vi "PID Movement final version.vi"(2 "error in (no error)":errorcluster, 3 "Yaw":dbl, 4 "Speed":dbl, 5 "Direction":T1) -> (0 "error out":errorcluster, 1 "Speed & distance":T2)   [LabVIEW 2018]
uses:
  PID Movement final version Type Def.ctl
  <vilib>/Studica/Studica Toolkit/Background/Mxp Selection.ctl
  <vilib>/addons/control/pid/pid.llb/PID (DBL).vi
  <vilib>/addons/control/pid/NI_PID_pid.lvlib
panel:
  out "Vx":dbl
  out "M2":dbl
  out "M1":dbl
  out "M0":dbl
  out "S2":dbl
  out "S1":dbl
  out "S0":dbl
  out "M2 Distance":dbl
  out "M1 Distance":dbl
  out "M0 Distance":dbl
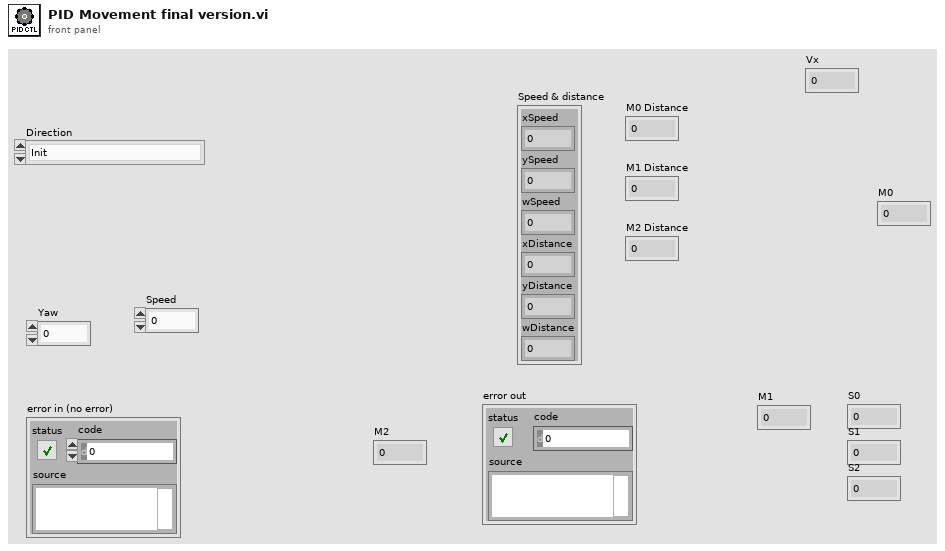
[diagram p1: front panel]
types:
  T1 = typedef "PID Movement final version Type Def.ctl" = enum16{"Init", "Front Back", "Left Right", "Rotate", "Latch", "Stop"}
  T2 = cluster{"xSpeed":dbl, "ySpeed":dbl, "wSpeed":dbl, "xDistance":dbl, "yDistance":dbl, "wDistance":dbl}
  T3 = cluster{"proportional gain (Kc)":dbl, "integral time (Ti, min)":dbl, "derivative time (Td, min)":dbl}
  T4 = typedef "Mxp Selection.ctl" = enum16{"MXP A", "MXP B"}
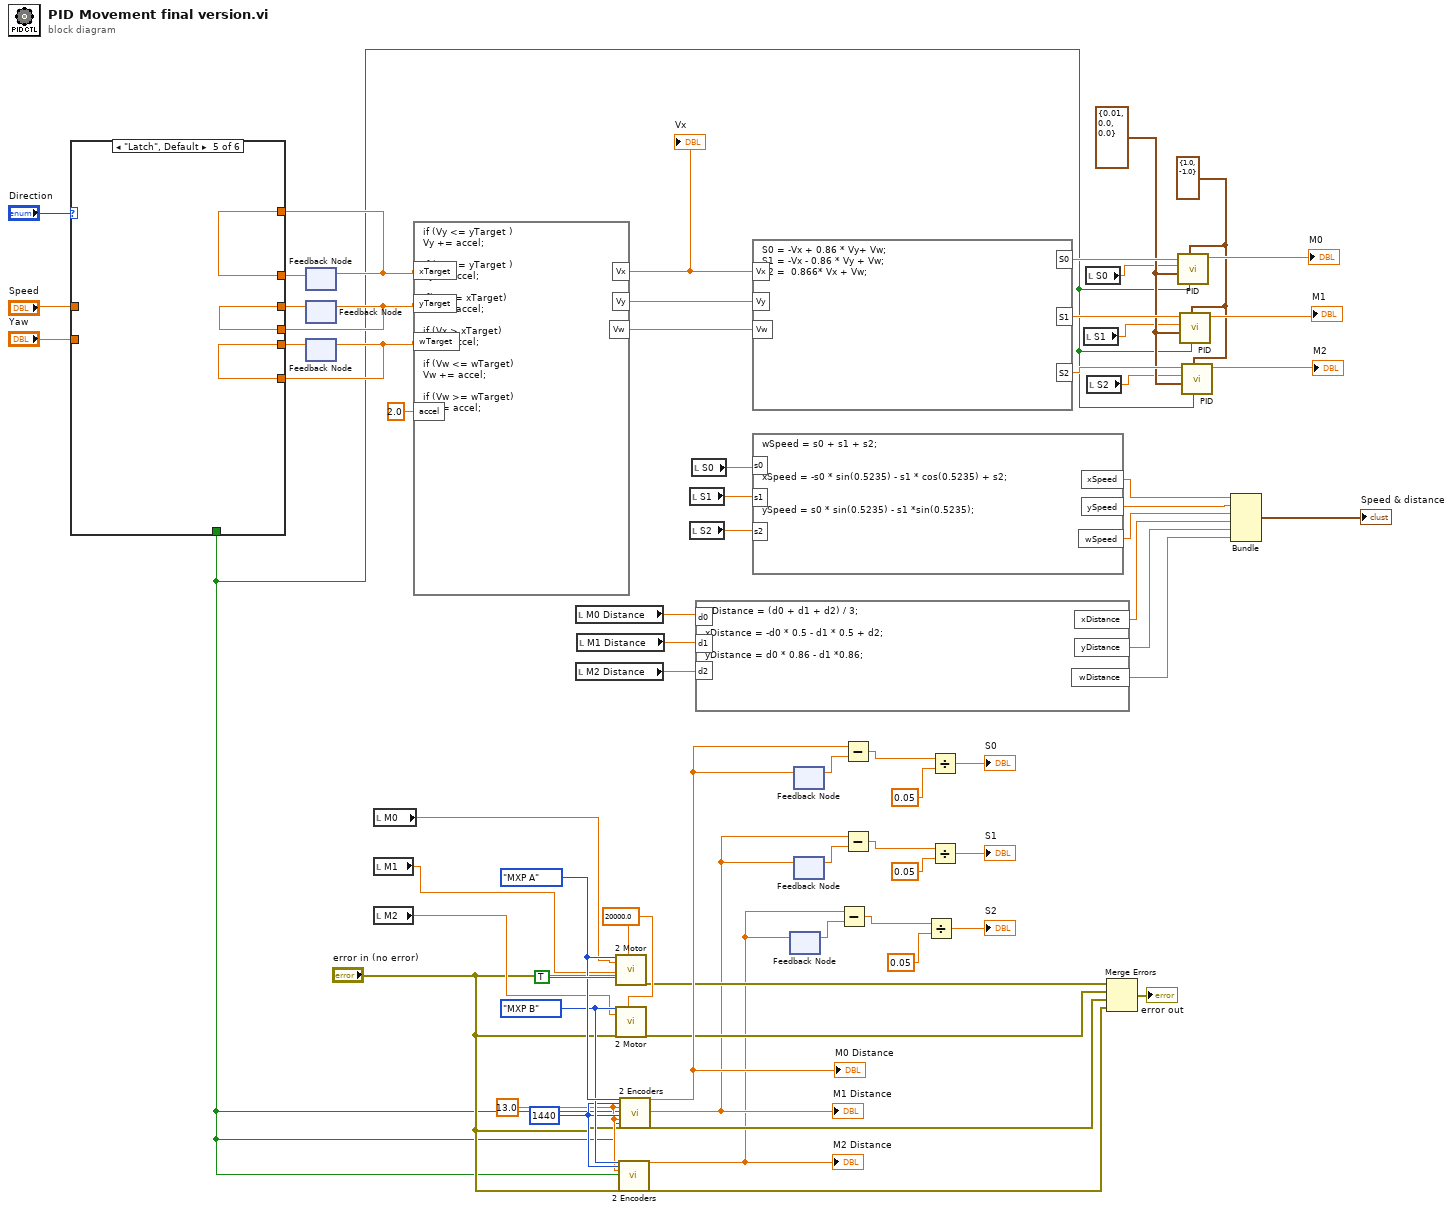
[diagram p0: block diagram]
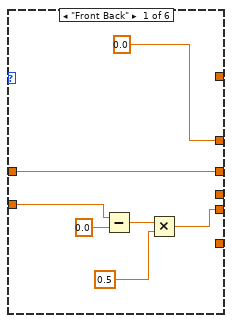
[diagram p2: hidden frame]
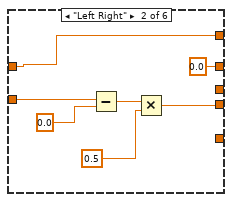
[diagram p3: hidden frame]
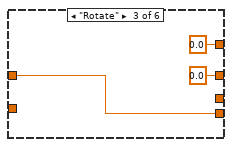
[diagram p4: hidden frame]
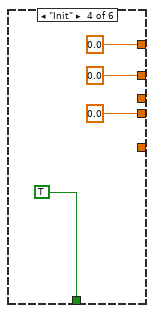
[diagram p5: hidden frame]
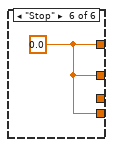
[diagram p6: hidden frame]
diagram:
  w6 = T3 {"proportional gain (Kc)"=0.01, "integral time (Ti, min)"=0.0, "derivative time (Td, min)"=0.0} ("PID gains")
  w5 = cluster{"output high":dbl, "output low":dbl} {"output high"=1.0, "output low"=-1.0} ("output range")
  w63 = 13.0 ("Wheel Diameter M0 (inches)")
  w64 = u32 1440 ("Ticks Per Rev M0")
  w68 = 20000.0 ("Frequency [Hz]")
  w66 = Mxp_Selection."MXP A" ("Mxp Side")
  w65 = Mxp_Selection."MXP B" ("Mxp Side")
  n1 = feedback #1() -> (w19:dbl)  [unwired: 1 in]
  n2 = feedback #2() -> (w18:dbl)  [unwired: 1 in]
  n3 = feedback #3() -> (w17:dbl)  [unwired: 1 in]
  n4 = case shown="\"Latch\", Default" "Direction" {
    tunnel: [0.0 w82 0.0 ("Speed") 0.0 w92 w93] -> w22
    tunnel: [w69 0.0 ("Speed") 0.0 ("Speed") 0.0 w91 w93] -> w21
    tunnel: [w71 w77 w83 0.0 w90 w93] -> w20
    tunnel: "Speed" -> [w69 w82 w83 _ _ _]
    tunnel: "Yaw" -> [w70 w76 _ _ _ _]
    tunnel: w19 -> [_ _ _ _ w92 _]
    tunnel: w18 -> [_ _ _ _ w91 _]
    tunnel: w17 -> [_ _ _ _ w90 _]
    tunnel: [_ _ _ TRUE ("Invert M1") _ _] -> w1
    frame "Front Back" {
      n5 = Subtract(x=w70, y=0.0) -> (x-y=w74:dbl)
      n6 = Multiply(x=w74, y=0.5) -> (x*y=w71:dbl)
    }
    frame "Left Right" {
      n7 = Subtract(x=w76, y=0.0) -> (x-y=w80:dbl)
      n8 = Multiply(x=w80, y=0.5) -> (x*y=w77:dbl)
    }
    frame "Rotate" {
    }
    frame "Init" {
    }
    frame "Latch", Default {
    }
    frame "Stop" {
      w93 = 0.0 ("Speed")
    }
  }
  n9 = feedback-in #1(w22) -> ()
  n10 = feedback-in #2(w21) -> ()
  n11 = feedback-in #3(w20) -> ()
  n12 = local read "M0"() -> (w42:dbl)
  n13 = local read "M1"() -> (w41:dbl)
  n14 = local read "M2"() -> (w40:dbl)
  n15 = formula code="if (Vy <= yTarget )\nVy += accel;\n\nif (Vy >= yTarget )\nVy -= accel;\n\nif(Vx <= xTarget)\nVx += accel;\n\nif (Vx > xTarget)\nVx -= accel;\n\nif (Vw <= wTarget)\nVw += accel;\n\nif (Vw >= wTarget)\nVw -= accel;"("xTarget"=w19, "yTarget"=w18, "wTarget"=w17, "accel"=2.0 ("input variable")) -> ("Vy"=w14:dbl, "Vx"=w15:dbl, "Vw"=w13:dbl)
  "Vx" <- w15
  n16 = local read "M0 Distance"() -> (w36:dbl)
  n17 = local read "M2 Distance"() -> (w34:dbl)
  n18 = local read "M1 Distance"() -> (w35:dbl)
  n19 = call <vilib>:"2 Motor.vi"("Mxp Side"=w66, "Speed M0"=w42, "Speed M1"=w41, "Invert M1"=TRUE, "error in (no error)"="error in (no error)", "Frequency [Hz]"=w68) -> ("error out"=w58:errorcluster)  [unwired: 13 in]
  n20 = call <vilib>:"2 Motor.vi"("Mxp Side"=w65, "Speed M0"=w40, "error in (no error)"="error in (no error)", "Frequency [Hz]"=w68) -> ("error out"=w57:errorcluster)  [unwired: 15 in]
  n21 = call <vilib>:"2 Encoders.vi"("Mxp Side"=w65, "Ticks Per Rev M0"=w64, "Wheel Diameter M0 (inches)"=w63, "Reset Encoder 0"=w1, "error in (no error)"="error in (no error)") -> ("Distance M0 (inches)"=w46:dbl, "error out"=w55:errorcluster)  [unwired: 20 in, 1 out]
  "M2 Distance" <- w46
  n22 = call <vilib>:"2 Encoders.vi"("Mxp Side"=w66, "Ticks Per Rev M0"=w64, "Wheel Diameter M0 (inches)"=w63, "Reset Encoder 0"=w1, "Ticks Per Rev M1"=w64, "Wheel Diameter M1 (inches)"=w63, "Reset Encoder 1"=w1, "error in (no error)"="error in (no error)") -> ("Distance M0 (inches)"=w61:dbl, "Distance M1 (inches)"=w50:dbl, "error out"=w56:errorcluster)  [unwired: 17 in]
  "M0 Distance" <- w61
  "M1 Distance" <- w50
  n23 = local read "S1"() -> (w38:dbl)
  n24 = local read "S2"() -> (w37:dbl)
  n25 = local read "S0"() -> (w39:dbl)
  n26 = formula code="wDistance = (d0 + d1 + d2) / 3;\n\nxDistance = -d0 * 0.5 - d1 * 0.5 + d2;\n\nyDistance = d0 * 0.86 - d1 *0.86;"("d0"=w36, "d1"=w35, "d2"=w34) -> ("xDistance"=w29:dbl, "wDistance"=w27:dbl, "yDistance"=w28:dbl)
  n27 = formula code="S0 = -Vx + 0.86 * Vy+ Vw;\nS1 = -Vx - 0.86 * Vy + Vw;\nS2 =  0.866* Vx + Vw;"("Vx"=w15, "Vy"=w14, "Vw"=w13) -> ("S0"=w12:dbl, "S1"=w11:dbl, "S2"=w10:dbl)
  n28 = formula code="wSpeed = s0 + s1 + s2;\n\n\nxSpeed = -s0 * sin(0.5235) - s1 * cos(0.5235) + s2;\n\n\nySpeed = s0 * sin(0.5235) - s1 *sin(0.5235);"("s0"=w39, "s1"=w38, "s2"=w37) -> ("xSpeed"=w33:dbl, "ySpeed"=w32:dbl, "wSpeed"=w31:dbl)
  n29 = feedback #4() -> (w48:dbl)  [unwired: 1 in]
  n30 = feedback-in #4(w46) -> ()
  n31 = feedback #5() -> (w60:dbl)  [unwired: 1 in]
  n32 = feedback-in #5(w61) -> ()
  n33 = feedback #6() -> (w52:dbl)  [unwired: 1 in]
  n34 = feedback-in #6(w50) -> ()
  n35 = Subtract(x=w46, y=w48) -> (x-y=w49:dbl)
  n36 = Subtract(x=w61, y=w60) -> (x-y=w62:dbl)
  n37 = Subtract(x=w50, y=w52) -> (x-y=w53:dbl)
  n38 = Divide(x=w49, y=0.05) -> (x/y=→"S2":dbl)
  n39 = Divide(x=w62, y=0.05) -> (x/y=→"S0":dbl)
  n40 = Divide(x=w53, y=0.05) -> (x/y=→"S1":dbl)
  n41 = local read "S1"() -> (w3:dbl)
  n42 = local read "S0"() -> (w4:dbl)
  n43 = local read "S2"() -> (w2:dbl)
  n44 = Merge Errors(w58, w57, w56, w55) -> (→"error out":errorcluster)
  n45 = call-poly <vilib>:"PID.vi"("reinitialize? (F)"=w1, "output range"=w5, "PID gains"=w6, "process variable"=w4, "setpoint"=w12) -> ("output"=→"M0":dbl)  [unwired: 5 in, 1 out]
  n46 = call-poly <vilib>:"PID.vi"("reinitialize? (F)"=w1, "output range"=w5, "PID gains"=w6, "process variable"=w3, "setpoint"=w11) -> ("output"=→"M1":dbl)  [unwired: 5 in, 1 out]
  n47 = call-poly <vilib>:"PID.vi"("reinitialize? (F)"=w1, "output range"=w5, "PID gains"=w6, "process variable"=w2, "setpoint"=w10) -> ("output"=→"M2":dbl)  [unwired: 5 in, 1 out]
  n48 = Bundle("xSpeed"=w33, "ySpeed"=w32, "wSpeed"=w31, "xDistance"=w29, "yDistance"=w28, "wDistance"=w27) -> (→"Speed & distance":T2)  [unwired: 1 in]
